vi "GetColor.vi"(8 "error in (no error)":errorcluster, 11 "overlay in":refnum<class "overlay.lvclass">) -> (0 "error out":errorcluster, 2 "color":u32(colorbox)=9868950, 3 "overlay out":refnum<class "overlay.lvclass">)   [LabVIEW 2009, in "overlay.lvclass"]
uses:
  overlay.lvclass
  overlay.lvclass/overlay.ctl
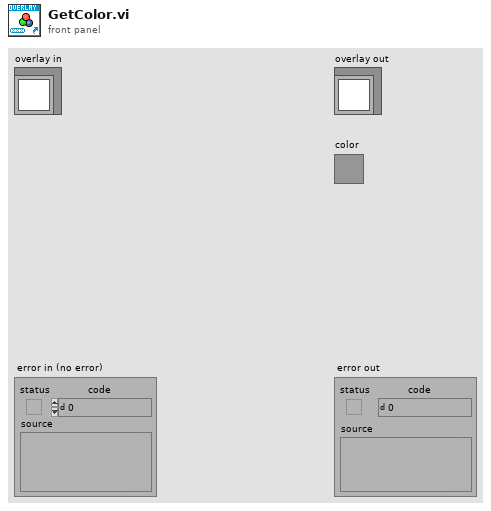
[diagram p1: front panel]
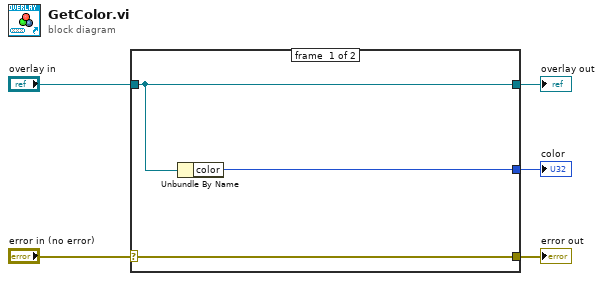
[diagram p0: block diagram]
diagram:
  n1 = case shown="No Error" "error in (no error)" {
    selector: "error in (no error)" -> [w8 w9]
    tunnel: [w8 w9] -> w2
    tunnel: [w7 w10] -> w4
    tunnel: "overlay in" -> [w7 w10]
    tunnel: [w6 _] -> w1
    frame #0 {
      n2 = Unbundle By Name(w7) -> ("color"=w6:u32)
    }
    frame #1 {
    }
  }
  "error out" <- w2
  "overlay out" <- w4
  "color" <- w1
